vi "LabVIEW Basics #5 - Radar Sweep.vi"() -> ()   [LabVIEW 2021]
uses:
  <vilib>/picture/picture.llb/imagedata.ctl
  <vilib>/Instr/_visa.llb/VISA Configure Serial Port (Instr).vi
panel:
  out "after substring":string
  out "before substring":string
  out "read buffer":string
  in  "stop":bool
  out "ping":bool
  out "Degrees":dbl format="%#_3f"
  out "Distance":dbl caption="CM" format="%#_2g"
  out "2D Picture":picture
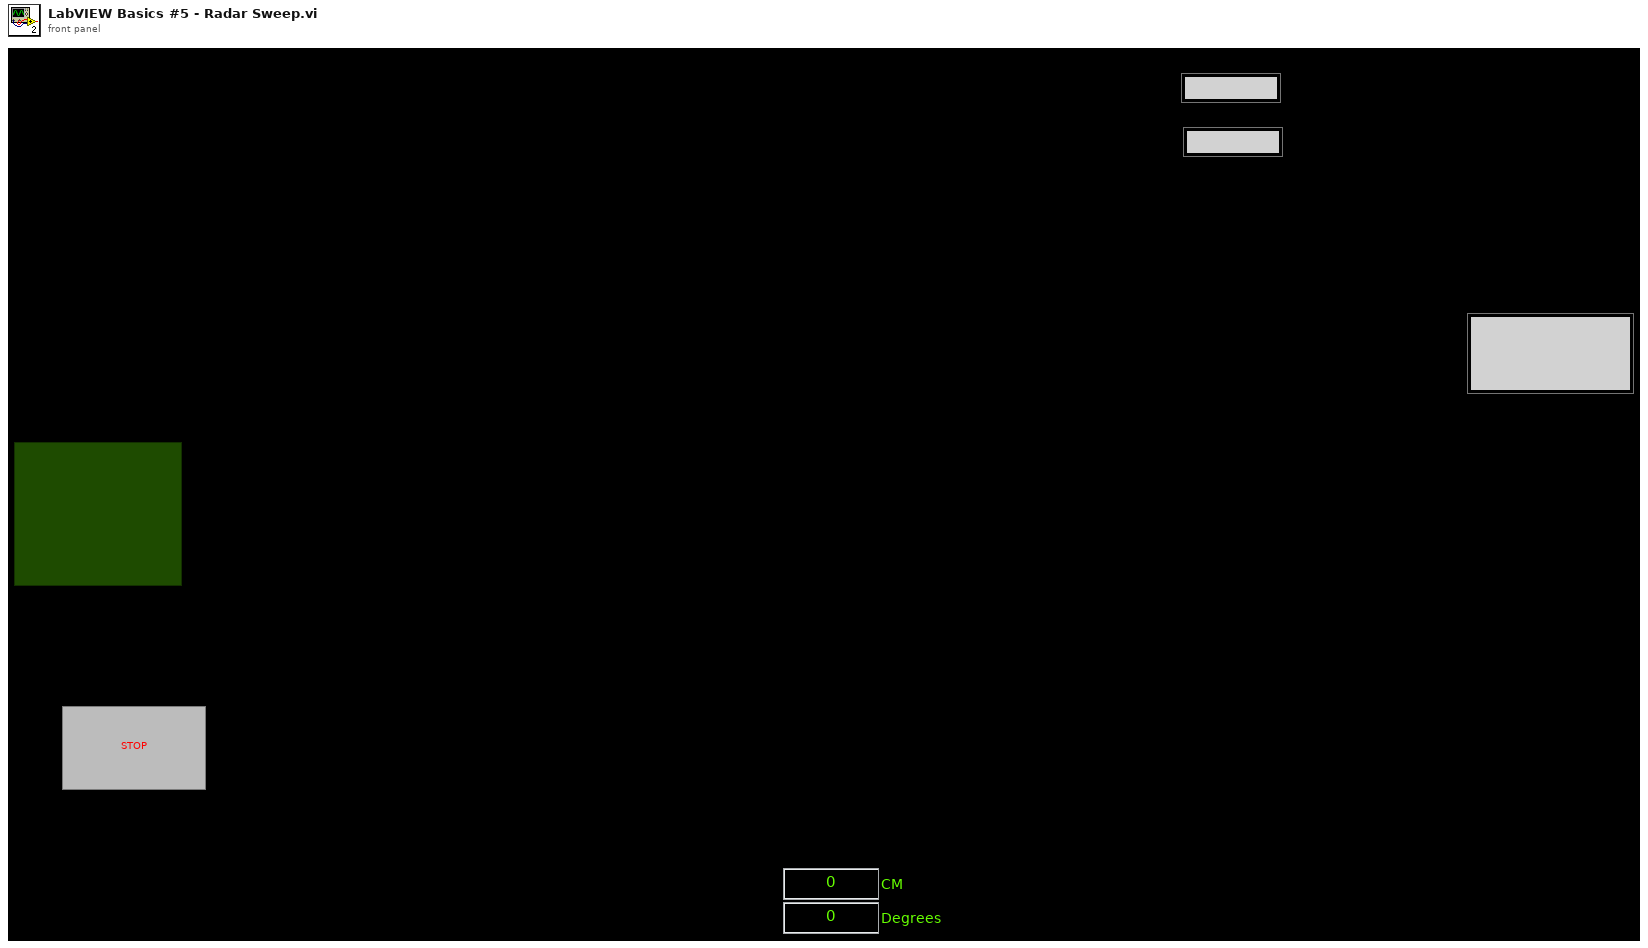
[diagram p1: front panel]
types:
  T1 = typedef "imagedata.ctl" = cluster{"image type":i32, "image depth":i32, "image":u8[], "mask":u8[], "colors":u32[], "Rectangle":cluster{"left":i16, "top":i16, "right":i16, "bottom":i16}}
  T2 = cluster{"maximum":dbl, "minimum":dbl, "clip to min":bool, "log?(F)":bool, "grid color":u32, "plot color":u32, "format and precision":cluster{"format":enum8{"Decimal", "Scientific", "Engineering", "Binary", "Octal", "Hex"}, "precision":u8}, "visible section":u16}
  T3 = typedef "LVBoundsTypeDef.ctl" = cluster{"Width":u32, "Height":u32}
  T4 = cluster{"pixel center":cluster{"x":i16, "y":i16}, "scale factors":cluster{"a":dbl, "b":dbl, "log?":bool}, "grid color":u32, "start angle":dbl, "end angle":dbl, "tick length":i16, "pixel radius":i32}
  T5 = cluster{"Distance (cm)":dbl, "Angle (Deg)":dbl}[]
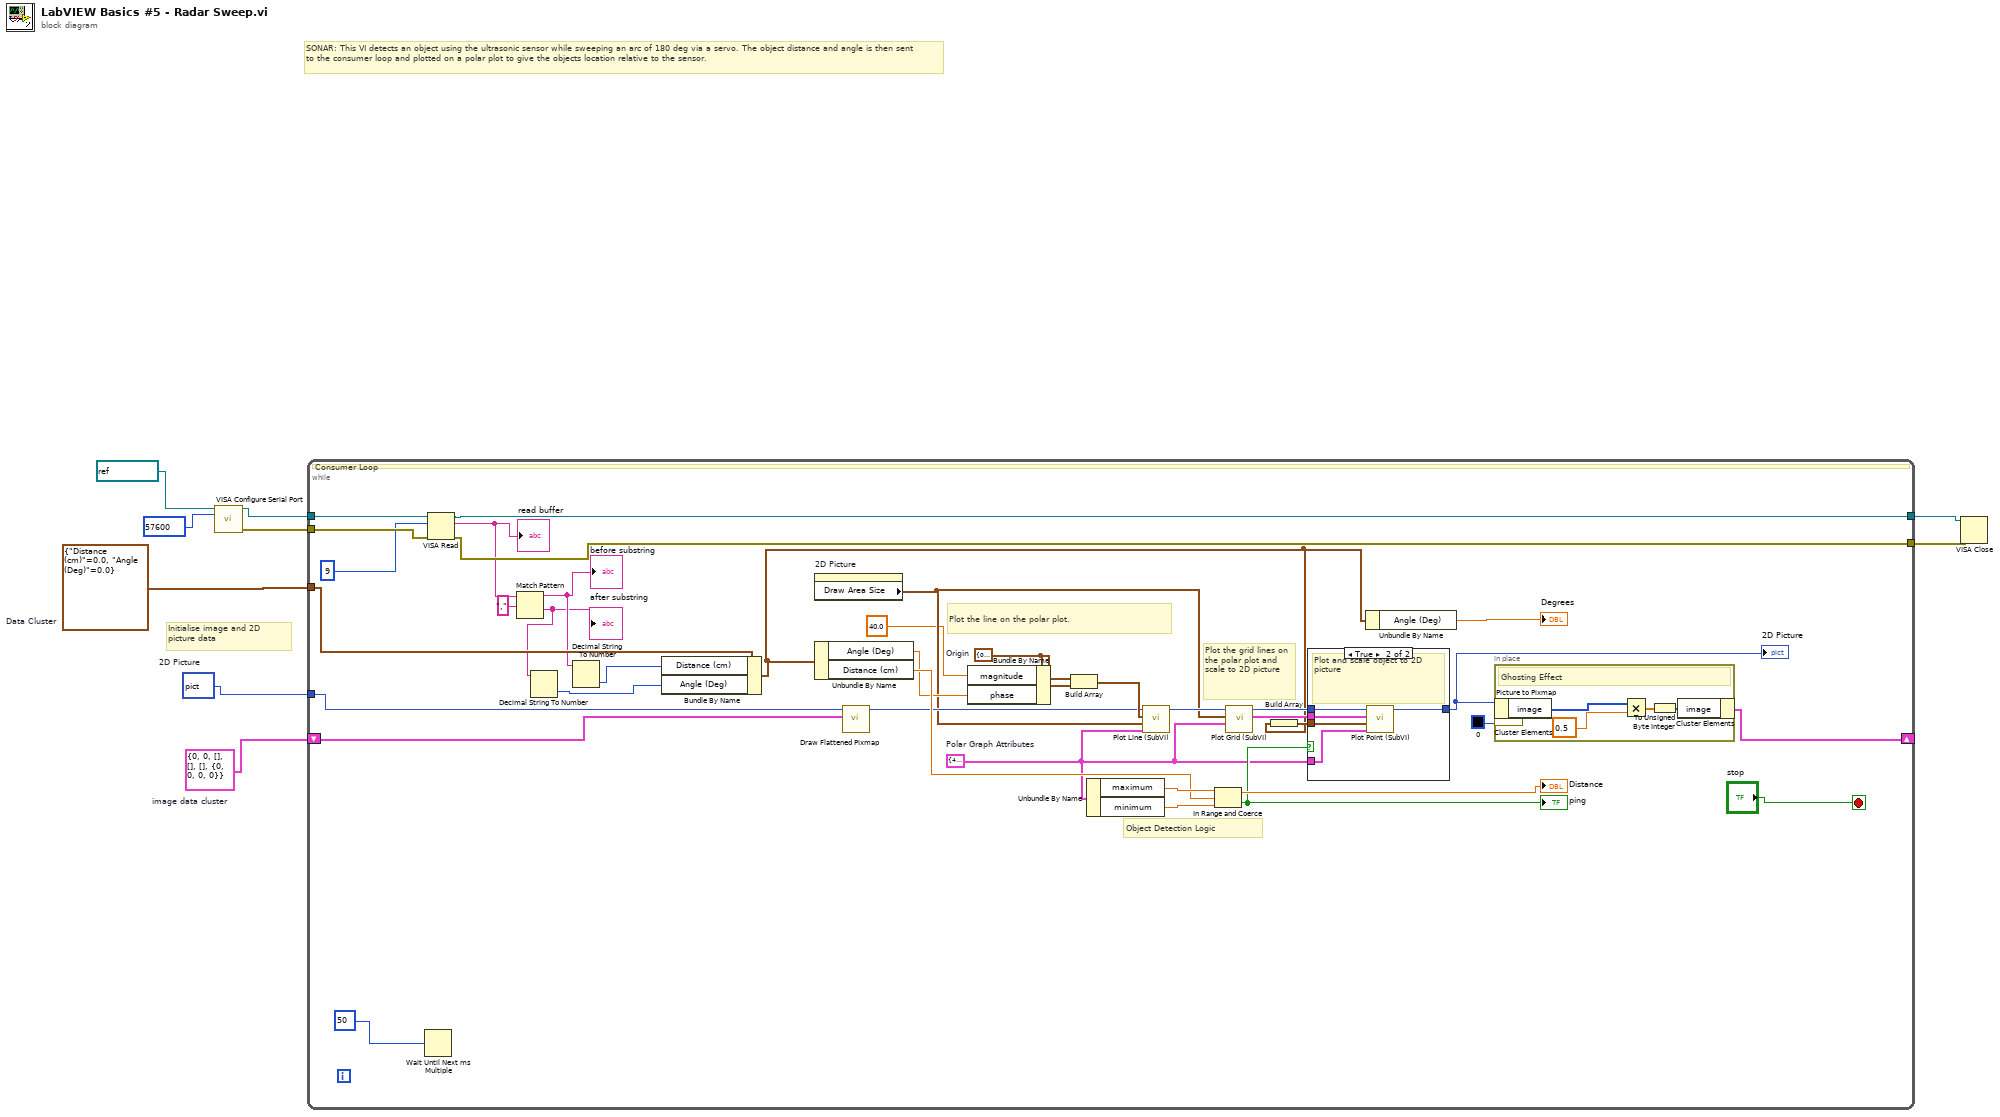
[diagram p0: block diagram]
diagram:
  w7 = cluster{"Distance (cm)":dbl, "Angle (Deg)":dbl} {"Distance (cm)"=0.0, "Angle (Deg)"=0.0}  # Data Cluster
  w8 = T1 {"image type"=0, "image depth"=0, "image"=[], "mask"=[], "colors"=[], "Rectangle"={"left"=0, "top"=0, "right"=0, "bottom"=0}}  # image data cluster
  w9 = picture data[5B]  # 2D Picture
  # "Initialise image and 2D picture data"
  # "SONAR: This VI detects an object using the ultrasonic sensor while sweeping an arc of 180 deg via a servo. The object distance and angle is then sent to the consumer loop and plotted on a polar plot to give the objects location relative to the sensor."
  n1 = call-poly "VISA Configure Serial Port"("VISA resource name"=refnum<visa-resource-name> "COM4", "baud rate (9600)"=u32 57600) -> ("VISA resource name out"=w6:refnum<visa-resource-name>, "error out"=w5:errorcluster)  [unwired: 12 in]
  n2 = while {
    tunnel: w9 -> [w48]
    shift-right: [w45] -> _
    shift-left: w8 -> [w47]
    tunnel: w7 -> [w24]
    tunnel: w6 -> [w20]
    tunnel: w5 -> [w19]
    tunnel: [w18] -> w3
    tunnel: [w17] -> w4
    stop <- "stop" stop-if-true
    w26 = cluster{"magnitude":dbl, "phase":dbl} {"magnitude"=0.0, "phase"=0.0}  # Origin
    w30 = T2 {"maximum"=40.0, "minimum"=2.0, "clip to min"=TRUE, "log?(F)"=FALSE, "grid color"=9868950, "plot color"=65280, "format and precision"={"format"=enum."Decimal", "precision"=0}, "visible section"=4}  # Polar Graph Attributes
    # "Object Detection Logic"
    # "Plot the line on the polar plot."
    # "Plot the grid lines on the polar plot and scale to 2D picture"
    # "Consumer Loop"
    n3 = Wait Until Next ms Multiple(millisecond multiple=50) -> ()  [unwired: 1 out]
    n4 = VISA Read(VISA resource name=w20, byte count=u32 9, error in (no error)=w19) -> (VISA resource name out=w17:refnum<visa-resource-name>, read buffer=w16:string, error out=w18:errorcluster)  [unwired: 1 out]
    "read buffer" <- w16
    n5 = Match Pattern(string=w16, regular expression=",") -> (before substring=w14:string, after substring=w12:string)  [unwired: 1 in, 2 out]
    "before substring" <- w14
    "after substring" <- w12
    n6 = Decimal String To Number(string=w12) -> (number=w11:i32)  [unwired: 2 in, 1 out]
    n7 = Decimal String To Number(string=w14) -> (number=w13:i32)  [unwired: 2 in, 1 out]
    n8 = Bundle By Name(cluster=w24, "Distance (cm)"=w13, "Angle (Deg)"=w11) -> (w23:cluster{"Distance (cm)":dbl, "Angle (Deg)":dbl})
    n9 = property on="2D Picture" class="Pict"() -> ("Draw Area Size"=w33:T3)  [unwired: 2 in, 2 out]
    n10 = Unbundle By Name(w23) -> ("Angle (Deg)"=w36:dbl, "Distance (cm)"=w37:dbl)
    n11 = call <vilib>:"Draw Flattened Pixmap.vi"("image data"=w47, "picture"=w48) -> ("new picture"=w34:picture)  [unwired: 7 in]
    n12 = Bundle By Name(cluster=w26, "magnitude"=40.0, "phase"=w36) -> (w25:cluster{"magnitude":dbl, "phase":dbl})
    n13 = Build Array(w26, w25) -> (w43:cluster{"magnitude":dbl, "phase":dbl}[])
    n14 = Unbundle By Name(w30) -> ("maximum"=w39:dbl, "minimum"=w38:dbl)
    n15 = call "Plot Line (SubVI).vi"("Polar Graph Attributes"=w30, "Draw Area Size"=w33, "Polar Array"=w43, "new picture in"=w34) -> ("new picture out"=w44:picture)  [unwired: 7 in]
    n16 = In Range and Coerce(upper limit=w39, x=w37, lower limit=w38) -> (coerced(x)=→"Distance":dbl, In Range?=w35:bool)
    "ping" <- w35
    n17 = call "Plot Grid (SubVI).vi"("Polar Graph Attributes"=w30, "Draw Area Size"=w33, "new picture in"=w44) -> ("grid measurements"=w41:T4, "new picture out"=w42:picture)  [unwired: 7 in]
    n18 = Build Array(w23) -> (w32:T5)
    n19 = case shown="True" w35 {
      tunnel: w32 -> [_ w54]
      tunnel: [w53 w58] -> w46
      tunnel: w42 -> [w53 w56]
      tunnel: w41 -> [_ w55]
      tunnel: w30 -> [_ w57]
      frame False {
        # "Nothing Detected"
      }
      frame True {
        # "Plot and scale object to 2D picture"
        n20 = call "Plot Point (SubVI).vi"("Polar Graph Attributes"=w57, "Array"=w54, "grid measurements"=w55, "new picture in"=w56) -> ("new picture"=w58:picture)  [unwired: 7 in]
      }
    }
    "2D Picture" <- w46
    n21 = Unbundle By Name(w23) -> ("Angle (Deg)"=→"Degrees":dbl)
    n22 = call <vilib>:"Picture to Pixmap.vi"("Background Color"=u32 0, "picture"=w46) -> ("image data"=w29:T1)  [unwired: 8 in, 1 out]
    n23 = in-place {
      # "Ghosting Effect"
      n24 = in-place-cluster #1(w29) -> ("image"=w52:u8[])
      n25 = Multiply(x=w52, y=0.5) -> (x*y=w50:dbl[])
      n26 = To Unsigned Byte Integer(number=w50) -> (unsigned 8bit integer=w49:u8[])
      n27 = in-place-cluster #1("image"=w49) -> (w45:T1)
    }
  }
  n28 = VISA Close(VISA resource name=w4, error in (no error)=w3) -> ()  [unwired: 1 out]
